vi "Generate Triggers (SubVI).vi"(10 "Bead Length Target":dbl, 11 "Cluster":cluster{dbl[], dbl[]}) -> (2 "Array":dbl[](array[numeric]), 3 "Array 2":cluster{dbl[], dbl[]}[](array[cluster]))   [LabVIEW 2016]
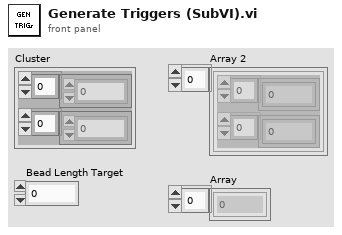
[diagram p1: front panel]
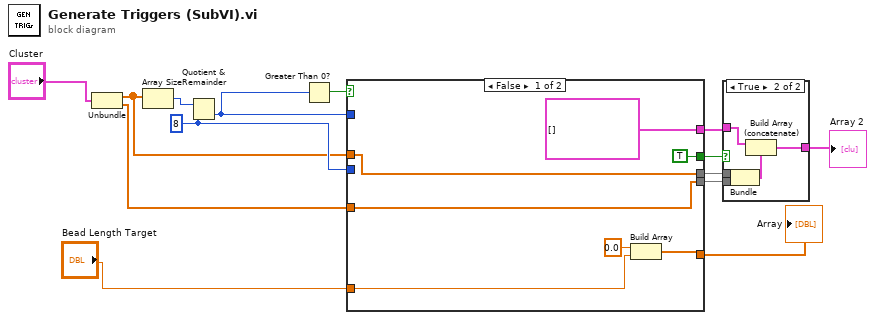
[diagram p0: block diagram]
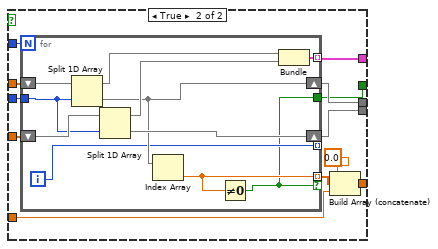
[diagram p2: hidden frame]
diagram:
  w7 = 8 ("y")
  n1 = Unbundle("Cluster") -> (w6:dbl[], w8:dbl[])
  n2 = Array Size(array=w6) -> (size(s)=w5:i32)
  n3 = Quotient & Remainder(x=w5, y=w7) -> (floor(x/y)=w2:i32)  [unwired: 1 out]
  n4 = Greater Than 0?(x=w2) -> (x > 0?=w1:bool)
  n5 = case shown="False" w1 {
    tunnel: "Bead Length Target" -> [w15 w33]
    tunnel: [w17 w32] -> w13
    tunnel: w2 -> [_ w29]
    tunnel: [w21 w28] -> w12
    tunnel: [cluster{dbl[], dbl[]}[] [] w27] -> w10
    tunnel: [w20 w26] -> w9
    tunnel: w8 -> [w20 w25]
    tunnel: w7 -> [_ w24]
    tunnel: w6 -> [w21 w23]
    tunnel: [TRUE w22] -> w3
    frame False {
      n6 = Build Array(0.0 ("element"), w15) -> (w17:dbl[])
    }
    frame True {
      n7 = for {
        N: w29 -> [_]
        tunnel: w24 -> [w38]
        shift-right: [w37] -> w28
        shift-left: w23 -> [w44]
        shift-right: [w41] -> w26
        shift-left: w25 -> [w43]
        tunnel: [w40] -> w27 mode=indexing
        tunnel: [w35] -> w31 mode=indexing if=w34
        tunnel: [w36] -> _ mode=indexing
        tunnel: [w34] -> w22
        i -> [w36]
        n8 = Split 1D Array(array=w44, index=w38) -> (first subarray=w42:dbl[], second subarray=w37:dbl[])
        n9 = Split 1D Array(array=w43, index=w38) -> (first subarray=w39:dbl[], second subarray=w41:dbl[])
        n10 = Index Array(array=w37) -> (element=w35:dbl)  [unwired: 1 in]
        n11 = Not Equal To 0?(x=w35) -> (x != 0?=w34:bool)
        n12 = Bundle(w42, w39) -> (w40:cluster{dbl[], dbl[]})  [unwired: 1 in]
      }
      n13 = Build Array (concatenate)(0.0, w31, w33) -> (w32:dbl[])
    }
  }
  "Array" <- w13
  n14 = case shown="True" w3 {
    tunnel: w12 -> [_ w50]
    tunnel: [w45 w49] -> w11
    tunnel: w10 -> [w45 w47]
    tunnel: w9 -> [_ w46]
    frame False {
    }
    frame True {
      n15 = Bundle(w50, w46) -> (w48:cluster{dbl[], dbl[]})  [unwired: 1 in]
      n16 = Build Array (concatenate)(w47, w48) -> (w49:cluster{dbl[], dbl[]}[])
    }
  }
  "Array 2" <- w11
